vi "Reserve Sessions.vi"(6 "timeout in milliseconds":i32, 8 "error in":errorcluster, 9 "instrument type ID":string, 10 "pin or relay names":string[](array[string]), 11 "Measurement Context In":refnum<class "MeasurementContext.lvclass">) -> (0 "error out":errorcluster, 1 "gRPC device location":T3, 2 "session information":T4[](array[typedef]), 3 "Measurement Context out":refnum<class "MeasurementContext.lvclass">, 5 "gRPC channel pool out":T1)   [LabVIEW 2020]
uses:
  <vilib>/MeasurementLink/MeasurementLink Session Management Client/RPC Messages/ni_measurementlink_sessionmanagement_v1_SessionInformation.ctl
  <vilib>/MeasurementLink/MeasurementLink Session Management Client/RPC Messages/nidevice_grpc_Session.ctl
  <vilib>/MeasurementLink/MeasurementLink Session Management Client/RPC Messages/ni_measurementlink_sessionmanagement_v1_ChannelMapping.ctl
  <vilib>/MeasurementLink/MeasurementLink Discovery Client/RPC Messages/ni_measurementlink_discovery_v1_ServiceLocation.ctl
  GRPC Channel Pool.ctl
  <vilib>/gRPC/LabVIEW gRPC Library/Shared/grpcId.ctl
  <vilib>/MeasurementLink/MeasurementLink Measurement Server/Classes/MeasurementContext/MeasurementContext.lvclass
  <vilib>/MeasurementLink/MeasurementLink Discovery Client/RPC Messages/ni_measurementlink_discovery_v1_ResolveServiceRequest.ctl
  <vilib>/MeasurementLink/MeasurementLink Session Management Client/RPC Messages/ni_measurementlink_sessionmanagement_v1_ReserveSessionsRequest.ctl
  <vilib>/MeasurementLink/MeasurementLink Session Management Client/RPC Messages/ni_measurementlink_PinMapContext.ctl
  <vilib>/MeasurementLink/MeasurementLink Measurement Server/MeasurementLink Measurement Server.lvlib
  <vilib>/MeasurementLink/MeasurementLink Discovery Client/MeasurementLink Discovery Client.lvlib
  <vilib>/MeasurementLink/MeasurementLink Session Management Client/MeasurementLink Session Management Client.lvlib
  NIDCPowerSourceDCVoltage.lvlib
  <vilib>/gRPC/LabVIEW gRPC Library/grpc-lvsupport-release.lvlib
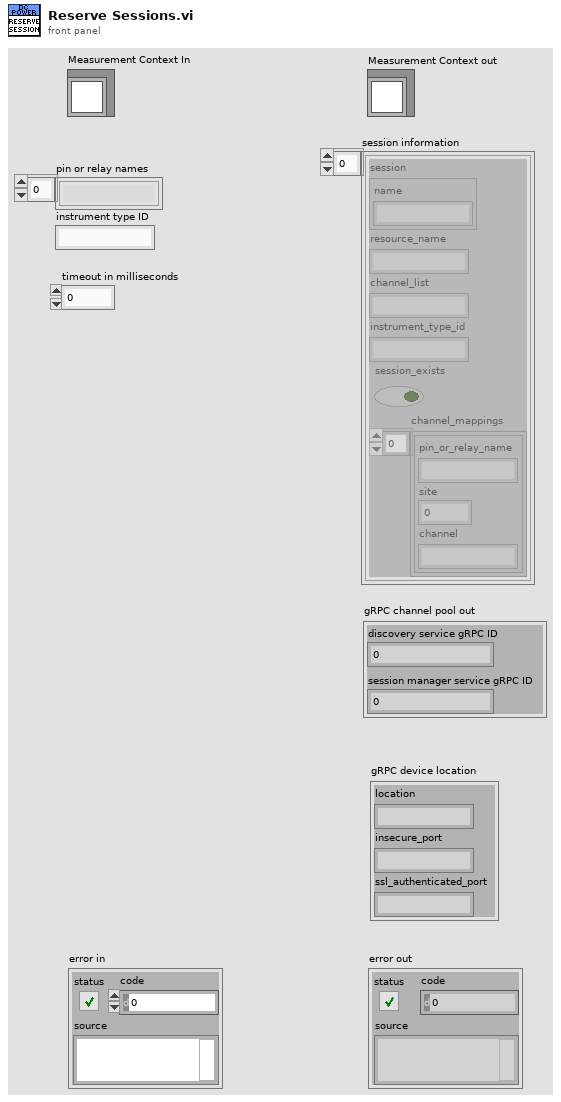
[diagram p1: front panel]
types:
  T1 = typedef "NIDCPowerSourceDCVoltage.lvlib/GRPC Channel Pool.ctl" = cluster{"discovery service gRPC ID":T2, "session manager service gRPC ID":T2}
  T2 = typedef "grpc-lvsupport-release.lvlib/grpcId.ctl" = u64
  T3 = typedef "MeasurementLink Discovery Client.lvlib/ni_measurementlink_discovery_v1_ServiceLocation.ctl" = cluster{"location":string, "insecure_port":string, "ssl_authenticated_port":string}
  T4 = typedef "MeasurementLink Session Management Client.lvlib/ni_measurementlink_sessionmanagement_v1_SessionInformation.ctl" = cluster{"session":T5, "resource_name":string, "channel_list":string, "instrument_type_id":string, "session_exists":bool, "channel_mappings":T6[]}
  T5 = typedef "MeasurementLink Session Management Client.lvlib/nidevice_grpc_Session.ctl" = cluster{"name":string}
  T6 = typedef "MeasurementLink Session Management Client.lvlib/ni_measurementlink_sessionmanagement_v1_ChannelMapping.ctl" = cluster{"pin_or_relay_name":string, "site":i32, "channel":string}
  T7 = typedef "MeasurementLink Session Management Client.lvlib/ni_measurementlink_sessionmanagement_v1_ReserveSessionsRequest.ctl" = cluster{"pin_map_context":T8, "pin_or_relay_names":string[], "instrument_type_id":string, "timeout_in_milliseconds":i32}
  T8 = typedef "MeasurementLink Session Management Client.lvlib/ni_measurementlink_PinMapContext.ctl" = cluster{"pin_map_id":string, "sites":i32[]}
  T9 = typedef "MeasurementLink Discovery Client.lvlib/ni_measurementlink_discovery_v1_ResolveServiceRequest.ctl" = cluster{"provided_interface":string, "service_class":string}
  T10 = typedef "MeasurementLink Measurement Server.lvlib/PinMapContext.ctl" = cluster{"pin_map_id":string, "sites":i32[]}
  T11 = typedef "MeasurementLink Session Management Client.lvlib/ni_measurementlink_sessionmanagement_v1_ReserveSessionsResponse.ctl" = cluster{"sessions":T4[]}
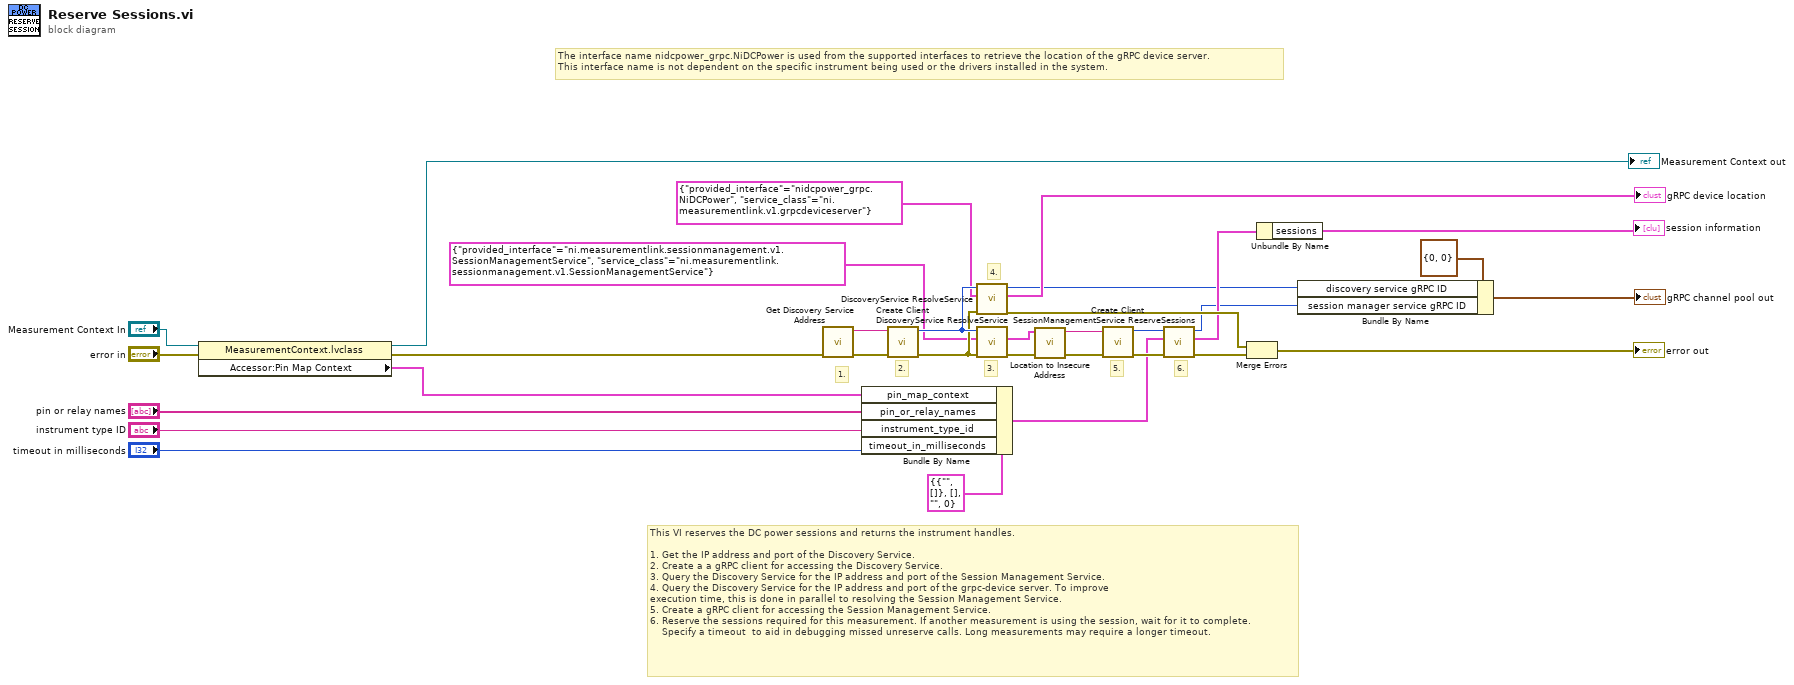
[diagram p0: block diagram]
diagram:
  # "The interface name nidcpower_grpc.NiDCPower is used from the supported interfaces to retrieve the location of the gRPC device server. \nThis interface name is not dependent on the specific instrument being used or the drivers installed in the system."
  # "6."
  # "5."
  # "4."
  # "3."
  # "2."
  # "1."
  # "This VI reserves the DC power sessions and returns the instrument handles.\n\n1. Get the IP address and port of the Discovery Service.\n2. Create a a gRPC client for accessing the Discovery Service.\n3. Query the Discovery Service for the IP address and port of the Session Management Service.\n4. Query the Discovery Service for the IP address and port of the grpc-device server. To improve \nexecution time, this is done in parallel to resolving the Session Management Service.\n5. Create a gRPC client for accessing the Session Management Service.\n6. Reserve the sessions required for this measurement. If another measurement is using the session, wait for it to complete. \n    Specify a timeout  to aid in debugging missed unreserve calls. Long measurements may require a longer timeout."
  n1 = property class="MeasurementContext.lvclass"(reference="Measurement Context In", error in="error in") -> (reference out=→"Measurement Context out":refnum<class "MeasurementContext.lvclass">, error out=w4:errorcluster, "Accessor:Pin Map Context"=w2:T10)
  n2 = call <vilib>:"Get Discovery Service Address.vi"("error in"=w4) -> ("error out"=w31:errorcluster, "address"=w30:string)  [unwired: 9 in]
  n3 = Bundle By Name(cluster=T7 {"pin_map_context"={"pin_map_id"="", "sites"=[]}, "pin_or_relay_names"=[], "instrument_type_id"="", "timeout_in_milliseconds"=0} ("Request Data"), "pin_map_context"=w2, "pin_or_relay_names"="pin or relay names", "instrument_type_id"="instrument type ID", "timeout_in_milliseconds"="timeout in milliseconds") -> (w14:T7)
  n4 = call <vilib>:"Create Client.vi"("error in"=w31, "address"=w30) -> ("error out"=w23:errorcluster, "gRPC ID Out"=w24:T2)  [unwired: 8 in]
  n5 = call <vilib>:"DiscoveryService ResolveService.vi"("error in"=w23, "Request Data"=T9 {"provided_interface"="nidcpower_grpc.NiDCPower", "service_class"="ni.measurementlink.v1.grpcdeviceserver"}, "gRPC ID"=w24) -> ("error out"=w26:errorcluster, "Response Data"=→"gRPC device location":T3, "gRPC ID out"=w8:T2)  [unwired: 6 in]
  n6 = call <vilib>:"DiscoveryService ResolveService.vi"("error in"=w23, "Request Data"=T9 {"provided_interface"="ni.measurementlink.sessionmanagement.v1.SessionManagementService", "service_class"="ni.measurementlink.sessionmanagement.v1.SessionManagementService"}, "gRPC ID"=w24) -> ("error out"=w27:errorcluster, "Response Data"=w10:T3)  [unwired: 6 in, 1 out]
  n7 = call "Location to Insecure Address.vi"("Response Data"=w10) -> ("String"=w9:string)  [unwired: 10 in]
  n8 = call <vilib>:"Create Client.vi"("error in"=w27, "address"=w9) -> ("error out"=w28:errorcluster, "gRPC ID Out"=w29:T2)  [unwired: 8 in]
  n9 = call <vilib>:"SessionManagementService ReserveSessions.vi"("error in"=w28, "Request Data"=w14, "gRPC ID"=w29) -> ("error out"=w25:errorcluster, "Response Data"=w20:T11, "gRPC ID out"=w7:T2)  [unwired: 6 in]
  n10 = Merge Errors(w26, w25) -> (→"error out":errorcluster)
  n11 = Unbundle By Name(w20) -> ("sessions"=→"session information":T4[])
  n12 = Bundle By Name(cluster=T1 {"discovery service gRPC ID"=0, "session manager service gRPC ID"=0} ("gRPC channel pool out"), "discovery service gRPC ID"=w8, "session manager service gRPC ID"=w7) -> (→"gRPC channel pool out":T1)
